vi "I2C Configure.vi"(8 "error in":errorcluster, 10 "I2C User Configuration":T1, 11 "FPGA VI Reference In":T2) -> (0 "error out":errorcluster, 3 "FPGA VI Reference Out":T2)   [LabVIEW 2015]
uses:
  DSDB FPGA Ref.ctl
  I2C User Configuration.ctl
  <vilib>/Utility/error.llb/Error Cluster From Error Code.vi
  <vilib>/rvi/errors/niLvFpgaAdjustHostInterfaceError.vi
  <vilib>/rvi/interface/nirviReadWriteControl/nirviReadWriteControl.xnode
  FPGA Bitfiles/Audio_FPGATarget_FPGAMain_3psOd07Wy8k.lvbitx
  FPGA Main.vi
  resource/NiAdept/NiAdept.dll
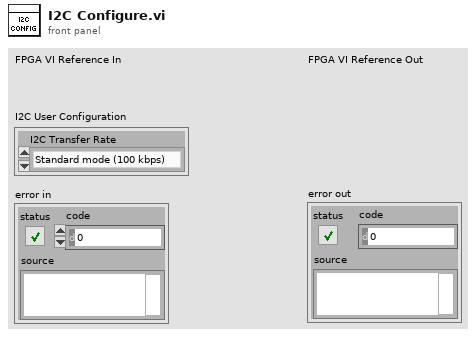
[diagram p1: front panel]
types:
  T1 = typedef "I2C User Configuration.ctl" = cluster{"I2C Transfer Rate":enum16{"Standard mode (100 kbps)", "Fast mode (400 kbps)"}}
  T2 = typedef "DSDB FPGA Ref.ctl" = refnum<k20>
  T3 = enum16{"Standard mode (100 kbps)", "Fast mode (400 kbps)"}
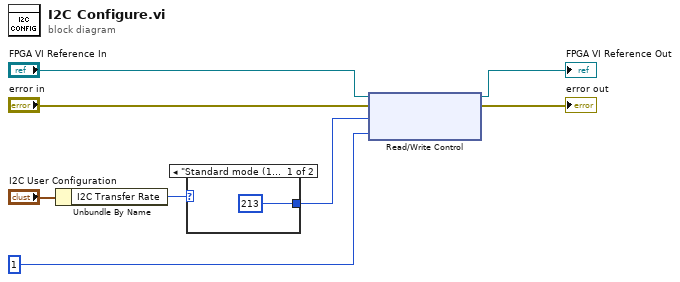
[diagram p0: block diagram]
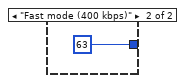
[diagram p2: hidden frame]
diagram:
  n1 = Unbundle By Name("I2C User Configuration") -> ("I2C Transfer Rate"=w1:T3)
  n2 = case shown="\"Standard mode (100 kbps)\", Default" w1 {
    tunnel: [u16 213 ("I2C.CNTR") u16 63 ("I2C.CNTR")] -> w4
    frame "Standard mode (100 kbps)", Default {
    }
    frame "Fast mode (400 kbps)" {
    }
  }
  n3 = xnode "Read/Write Control"("FPGA VI Reference In"="FPGA VI Reference In", "error in"="error in", "I2C.Counter"=w4, "I2C.Configuration"=u8 1 ("I2C.CNFG")) -> ("FPGA VI Reference Out"=→"FPGA VI Reference Out":T2, "error out"=→"error out":errorcluster)
